vi "NT Write Boolean Array.vi"(8 "error in":errorcluster, 9 "Boolean Array":bool[](array[boolean]), 11 "Name":string="Boolean Array") -> (0 "error out":errorcluster)   [LabVIEW 2017]
doc: "Write the Boolean array to the named entry."
uses:
  <vilib>/Rock Robotics/Network Tables/Field Data.ctl
  <vilib>/Rock Robotics/Network Tables/Field Type.ctl
  <vilib>/Rock Robotics/Network Tables/Sequence.ctl
  <vilib>/Rock Robotics/Network Tables/Write Value Core.vi
  <vilib>/Rock Robotics/Network Tables/Cached Name Lookup.vi
  <vilib>/Rock Robotics/Network Tables/Create Actual Table Name.vi
  <vilib>/Rock Robotics/Network Tables/Manage Dirty Field ID List.vi
  <vilib>/Rock Robotics/Network Tables/NT Globals.vi
  <vilib>/Rock Robotics/Network Tables/Update Other Clients.vi
  <vilib>/Rock Robotics/Network Tables/Build Entry Assign Buffer.vi
  <vilib>/Rock Robotics/Network Tables/Field Data Manager.vi
  <vilib>/Rock Robotics/Network Tables/Usage Statistics.vi
  <vilib>/Rock Robotics/Network Tables/Table Manager.vi
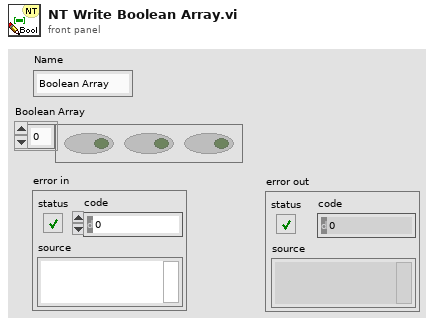
[diagram p1: front panel]
types:
  T1 = typedef "Field Data.ctl" = cluster{"Dbl":dbl, "String":string, "Type":T2, "Boolean":bool, "Sequence #":T3, "Flags":u8}
  T2 = typedef "Field Type.ctl" = enum8{"Invalid", "Bool", "Numeric", "String", "Raw", "Boolean Array", "Numeric Array", "String Array", "RPC"}
  T3 = typedef "Sequence.ctl" = u16
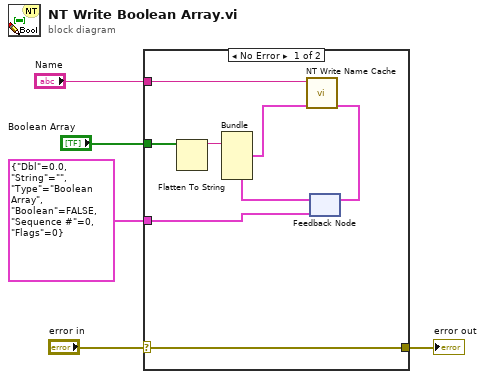
[diagram p0: block diagram]
diagram:
  n1 = case shown="No Error" "error in" {
    selector: "error in" -> [w6 w14]
    tunnel: "Boolean Array" -> [w13 _]
    tunnel: "Name" -> [w10 _]
    tunnel: T1 {"Dbl"=0.0, "String"="", "Type"=enum."Boolean Array", "Boolean"=FALSE, "Sequence #"=0, "Flags"=0} ("Field Value In") -> [w8 _]
    tunnel: [w6 w14] -> w1
    frame No Error {
      n2 = Flatten To String(anything=w13) -> (data string=w12:string)  [unwired: 3 in, 2 out]
      n3 = feedback #1(w8) -> (w7:T1)
      n4 = Bundle(cluster=w7, "String"=w12) -> (w11:T1)  [unwired: 5 in]
      n5 = call <vilib>:"NT Write Name Cache.vi"("Field Value In"=w11, "Name"=w10) -> ("Field Value Out"=w9:T1)  [unwired: 9 in]
      n6 = feedback-in #1(w9) -> ()
    }
    frame Error {
    }
  }
  "error out" <- w1
